vi "HCC Read Washer Config File.vi"(0 "Station and Board IDs":path, 2 "Configuration Path":path, 5 "Error In":errorcluster) -> (8 "Status Output Locations":path[](array[path])=[path "C:/Newfi Exe/Exe1/Configuration Files/Newfi Configuration.ini", path "C:/Newfi Exe/Exe2/Configuration Files/Newfi Configuration.ini", path "C:/Newfi Exe/Exe3/Configuration Files/Newfi Configuration.ini", path "C:/Newfi Exe/Exe4/Configuration Files/Newfi Configuration.ini", path "C:/Newfi Exe/Exe5/Configuration Files/Newfi Configuration.ini", path "C:/Newfi Exe/Exe6/Configuration Files/Newfi Configuration.ini", path "C:/Newfi Exe/Exe7/Configuration Files/Newfi Configuration.ini", path "C:/Newfi Exe/Exe8/Configuration Files/Newfi Configuration.ini", path "C:/Newfi Exe/Exe9/Configuration Files/Newfi Configuration.ini", path "C:/Newfi Exe/Exe10/Configuration Files/Newfi Configuration.ini", path "C:/Newfi Exe/Exe11/Configuration Files/Newfi Configuration.ini", path "C:/Newfi Exe/Exe12/Configuration Files/Newfi Configuration.ini", path "C:/Newfi Exe/Exe13/Configuration Files/Newfi Configuration.ini", path "C:/Newfi Exe/Exe14/Configuration Files/Newfi Configuration.ini", path "C:/Newfi Exe/Exe15/Configuration Files/Newfi Configuration.ini", path "C:/Newfi Exe/Exe16/Configuration Files/Newfi Configuration.ini", path "C:/Newfi Exe/Exe17/Configuration Files/Newfi Configuration.ini", path "C:/Newfi Exe/Exe18/Configuration Files/Newfi Configuration.ini", path "C:/Newfi Exe/Exe19/Configuration Files/Newfi Configuration.ini", path "C:/Newfi Exe/Exe20/Configuration Files/Newfi Configuration.ini", path "C:/Newfi Exe/Exe21/Configuration Files/Newfi Configuration.ini", path "C:/Newfi Exe/Exe22/Configuration Files/Newfi Configuration.ini", path "C:/Newfi Exe/Exe23/Configuration Files/Newfi Configuration.ini", path "C:/Newfi Exe/Exe24/Configuration Files/Newfi Configuration.ini"], 11 "Station IDs":string[](array[string])=["2M1", "2M2", "2M3", "2M4", "2M5", "2M6", "2M7", "2M8", "2M9", "2M10", "2M11", "2M12", "2M13", "2M14", "2M15", "2M16", "2M17", "2M18", "2M19", "2M20", "N/A", "N/A", "N/A", "N/A"], 13 "Voltage Indexes":i32[](array[numeric]), 14 "34972A_1":refnum<visa-resource-name>, 15 "34972A_2":refnum<visa-resource-name>, 16 "Board ID's":string[](array[string])=["", "", "", "", "", "", "", "", "", "", "", "", "7200002F", "72000040", "72000036", "7200003F", "7200003E", "72000387", "7200002E", "72000035", "", "", "", ""], 17 "Disable Channel = True":bool[](array[boolean])=[TRUE, TRUE, TRUE, TRUE, TRUE, TRUE, TRUE, TRUE, TRUE, TRUE, TRUE, TRUE, FALSE, FALSE, FALSE, FALSE, FALSE, FALSE, FALSE, FALSE, TRUE, TRUE, TRUE, TRUE], 18 "Agilent Channels DAQ":string="213,214,215,216,217,218,219,220", 19 "Error Out":errorcluster)   [LabVIEW 2016]
uses:
  <vilib>/Utility/file.llb/Read Delimited Spreadsheet (string).vi
panel:
  out "all rows":string[][](array[string])=[["Agilent Alias", "AGILENT236", ""], ["Current Transducer Type", " 1", ""], ["2M1", "", ""], ["2M2", "", ""], ["2M3", "", ""], ["2M4", "", ""], ["2M5", "", ""], ["2M6", "", ""], ["2M7", "", ""], ["2M8", "", ""], ["2M9", "", ""], ["2M10", "", ""], ["2M11", "", ""], ["2M12", "", ""], ["2M13", "7200002F", "213"], ["2M14", "72000040", "214"], ["2M15", "72000036", "215"], ["2M16", "7200003F", "216"], ["2M17", "7200003E", "217"], ["2M18", "72000387", "218"], ["2M19", "7200002E", "219"], ["2M20", "72000035", "220"], ["N/A", "", ""], ["N/A", "", ""], ["N/A", "", ""], ["N/A", "", ""]]
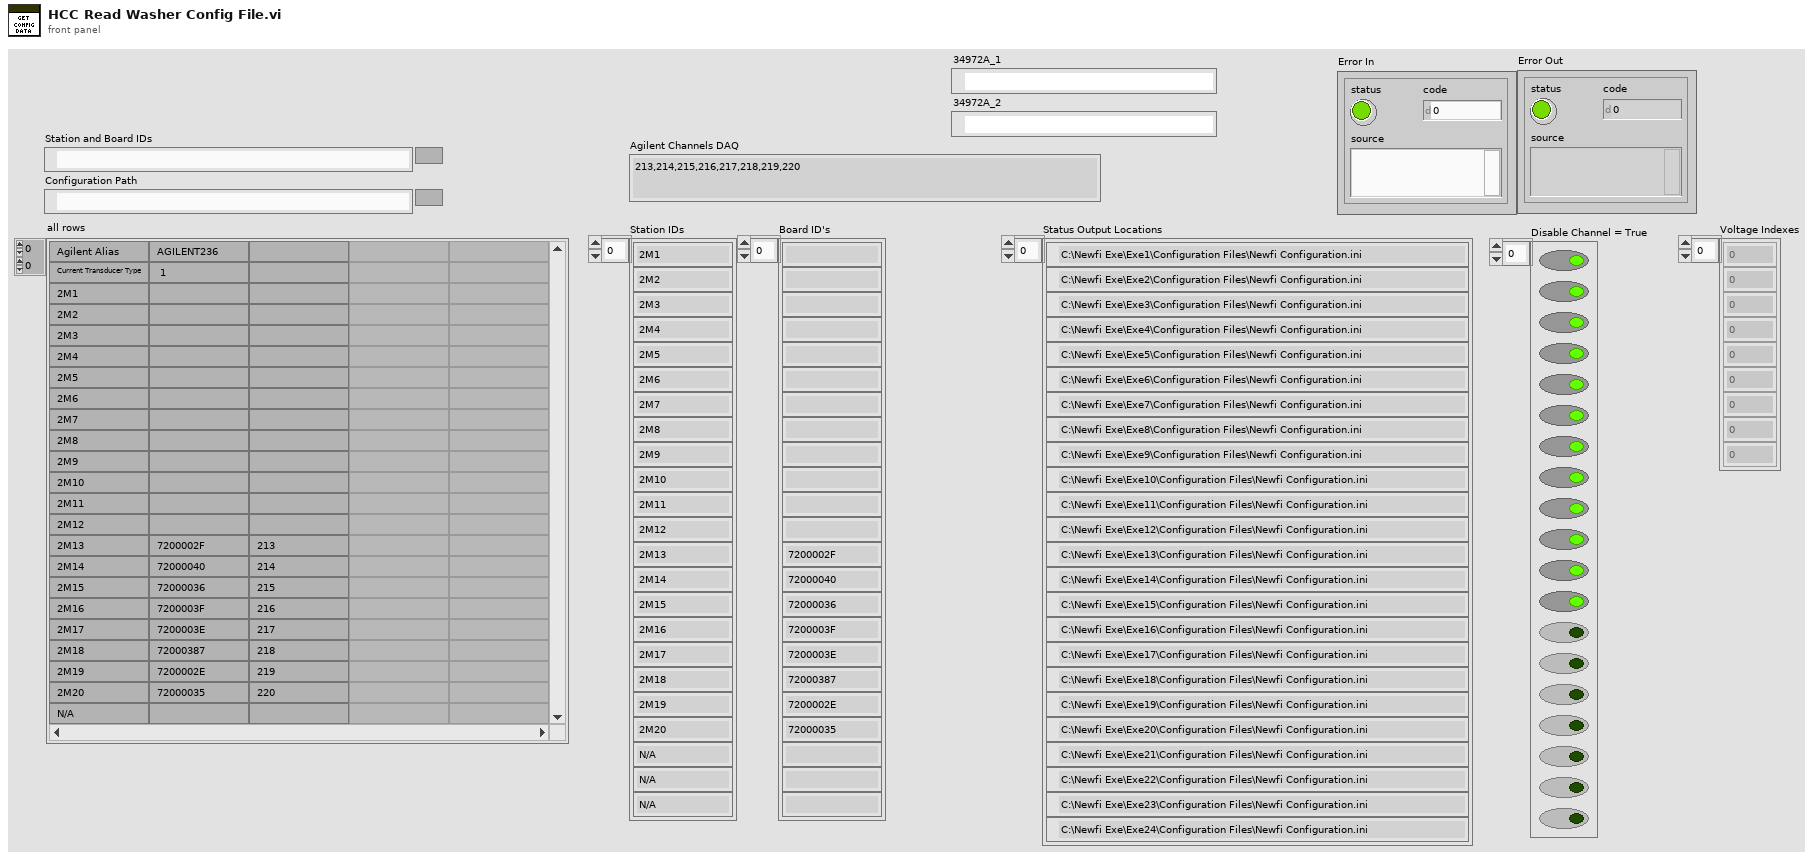
[diagram p1: front panel]
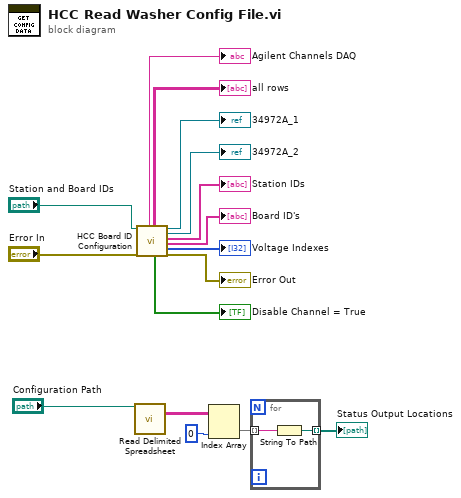
[diagram p0: block diagram]
diagram:
  n1 = call-poly <vilib>:"Read Delimited Spreadsheet.vi"("file path (dialog if empty)"="Configuration Path") -> ("all rows"=w1:string[][])  [unwired: 9 in, 5 out]
  n2 = call "HCC Board ID Configuration.vi"("Station and Board IDs"="Station and Board IDs", "Error In"="Error In") -> ("Agilent Channels DAQ"=→"Agilent Channels DAQ":string, "all rows"=→"all rows":string[][], "Disable Channel = True"=→"Disable Channel = True":bool[], "34972A_1"=→"34972A_1":refnum<visa-resource-name>, "34972A_2"=→"34972A_2":refnum<visa-resource-name>, "Station IDs"=→"Station IDs":string[], "Board ID's"=→"Board ID's":string[], "Voltage Indexes"=→"Voltage Indexes":i32[], "Error Out"=→"Error Out":errorcluster)  [unwired: 9 in]
  n3 = Index Array(array=w1, index (col)=0 ("disabled index (col)")) -> (element=w14:string[])  [unwired: 1 in]
  n4 = for {
    tunnel: w14 -> [w18] mode=indexing
    tunnel: [w17] -> w15 mode=indexing
    n5 = String To Path(string=w18) -> (path=w17:path)
  }
  "Status Output Locations" <- w15
